vi "Get Value.vi"(11 "AO in":refnum<class "AO.lvclass">) -> (2 "Value":dbl)   [LabVIEW 2019, in "AO.lvclass"]
uses:
  AO.lvclass
  AO.lvclass/AO.ctl
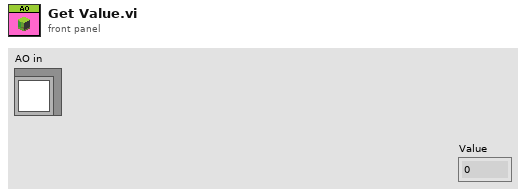
[diagram p1: front panel]
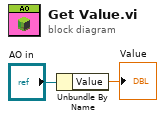
[diagram p0: block diagram]
diagram:
  n1 = Unbundle By Name("AO in") -> ("Value"=→"Value":dbl)
